vi "Begin.vi"(8 "error in":errorcluster) -> (0 "error out":errorcluster)   [LabVIEW 2019]
doc: "Called before other user functions, this VI is expected to open initial I/O refnums, load in file data, and do all program initialization. Notice that the <B>error out</B> terminal is simply used for data flow. Wiring it to other structures or subVIs ensures that this VI runs first."
uses:
  <vilib>/Rock Robotics/WPI/DriverStation/WPI_DriverStationRobotMode2.ctl
  <vilib>/Rock Robotics/WPI/Joystick/WPI_JoystickDeviceEnum.ctl
  <vilib>/Rock Robotics/SystemInterfaces/DIO/FPGA_DIOPWMChannel.ctl
  <vilib>/Rock Robotics/SystemInterfaces/DIO/FPGA_DIOChannel.ctl
  <vilib>/Rock Robotics/WPI/Solenoid/WPI_SolenoidChannel.ctl
  <vilib>/Rock Robotics/WPI/Accelerometer/WPI_AccelerometerAnalogChannels.ctl
  <vilib>/Rock Robotics/SystemInterfaces/AI/FPGA_AIChannel.ctl
  Robot Global Data.vi
  <vilib>/Rock Robotics/WPI/MotorControl/WPI_MotorControlOpen SPARK.vi
  <vilib>/Rock Robotics/WPI/Solenoid/WPI_SolenoidOpenDouble.vi
  <vilib>/Rock Robotics/WPI/Accelerometer/WPI_AccelerometerAnalogOpen.vi
  <vilib>/Rock Robotics/WPI/Switch/WPI_SwitchOpenLimit.vi
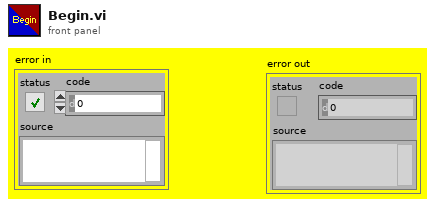
[diagram p1: front panel]
types:
  T1 = typedef "FPGA_DIOChannel.ctl" = enum8{"DIO 0", "DIO 1", "DIO 2", "DIO 3", "DIO 4", "DIO 5", "DIO 6", "DIO 7", "DIO 8", "DIO 9", "DIO MXP 0", "DIO MXP 1", "DIO MXP 2", "DIO MXP 3", "DIO MXP 4", "DIO MXP 5", "DIO MXP 6", "DIO MXP 7", "DIO MXP 8", "DIO MXP 9", "DIO MXP 10", "DIO MXP 11", "DIO MXP 12", "DIO MXP 13", "DIO MXP 14", "DIO MXP 15", "SPI Port CS1", "SPI Port CS2", "SPI Port CS3", "SPI Port MISO", "SPI Port MOSI", "Invalid"}
  T2 = typedef "FPGA_AIChannel.ctl" = enum8{"AI 0", "AI 1", "AI 2", "AI 3", "AI MXP 0", "AI MXP 1", "AI MXP 2", "AI MXP 3", "Invalid"}
  T3 = typedef "WPI_SolenoidChannel.ctl" = enum8{"Solenoid 0", "Solenoid 1", "Solenoid 2", "Solenoid 3", "Solenoid 4", "Solenoid 5", "Solenoid 6", "Solenoid 7", "Invalid"}
  T4 = typedef "WPI_AccelerometerAnalogChannels.ctl" = cluster{"X-Axis":T2, "Y-Axis":T2, "Z-Axis":T2}
  T5 = typedef "FPGA_DIOPWMChannel.ctl" = enum8{"PWM 0", "PWM 1", "PWM 2", "PWM 3", "PWM 4", "PWM 5", "PWM 6", "PWM 7", "PWM 8", "PWM 9", "PWM MXP 0", "PWM MXP 1", "PWM MXP 2", "PWM MXP 3", "PWM MXP 4", "PWM MXP 5", "PWM MXP 6", "PWM MXP 7", "PWM MXP 8", "PWM MXP 9", "Invalid"}
  T6 = typedef "WPI_JoystickDeviceEnum.ctl" = enum16{"USB 0", "USB 1", "USB 2", "USB 3", "USB 4", "USB 5"}
  T7 = typedef "WPI_DriverStationRobotMode2.ctl" = enum16{"Autonomous Disabled", "Autonomous Enabled", "Teleop Disabled", "Teleop Enabled", "Disconnected", "Finish", "Test Disabled", "Test Enabled", "Emergency Stopped"}
  T8 = typedef "WPI_JoystickDevRef.ctl" = cluster{"Device":T6}
  T9 = typedef "WPI_DigitalOutputDevRef.ctl" = cluster{"DIO Channel":T1, "DevStatus":errorcluster}
  T10 = typedef "WPI_MotorControlDeviceRef.ctl" = cluster{"DeviceStatus":errorcluster, "Type":T11, "PWM":cluster{"PWM Channel":T5, "DeadBand":T12}, "CAN":cluster{"Device Number":u8, "SetOutput VI Ref":variant, "GetOutput VI Ref":variant, "Enable VI Ref":variant, "Disable VI Ref":variant, "Data":variant}, "Invert":bool, "DIO PWM":cluster{"PWM \"Enable\" Channel":T5, "DIOChannel":T1, "PWM Rate":dbl}}
  T11 = typedef "WPI_MotorControlType.ctl" = enum16{"PWM", "CAN", "DIO PWM"}
  T12 = typedef "WPI_PWMDeadband.ctl" = cluster{"Name":string, "maxPositivePwm":i32, "minPositivePwm":i32, "centerPwm":i32, "maxNegativePwm":i32, "minNegativePwm":i32, "angularRange":u16}
  T13 = typedef "WPI_SolenoidDevRef.ctl" = cluster{"DevStatus":errorcluster, "Pneumatics Control Module":u8, "Forward Solenoid Channel":T3, "Reverse Solenoid Channel":T3}
  T14 = typedef "WPI_SwitchDevRef.ctl" = cluster{"DevStatus":errorcluster, "DIO Channel":T1, "CntIndex":T15, "Normally Closed":bool}
  T15 = typedef "FPGA_CounterCtrSystemIndex.ctl" = enum8{"Ctr 0", "Ctr 1", "Ctr 2", "Ctr 3", "Ctr 4", "Ctr 5", "Ctr 6", "Ctr 7", "Invalid"}
  T16 = typedef "WPI_PotentiometerDevRef.ctl" = cluster{"DevStatus":errorcluster, "Analog Channel":T2, "Invert Output":bool}
  T17 = typedef "WPI_AccelerometerDevRef.ctl" = cluster{"DevStatus":errorcluster, "Scaling":T18, "Analog Channels":T4, "I2C Bus":T19, "SPI Bus":T20, "Accel Range":T21, "ADXL Axes":T22, "Handle":i32, "Device Address":u8, "Accel Type":enum16{"Analog", "ADXL345 I2C", "ADXL345 SPI", "Internal", "ADXL362 SPI"}}
  T18 = typedef "WPI_AccelerometerScaling.ctl" = cluster{"Gain (VoltsPerG)":dbl, "Center Voltage":dbl}
  T19 = typedef "i2c_bus.ctl" = enum16{"I2C On-Board", "I2C MXP", "Invalid"}
  T20 = typedef "spi_bus.ctl" = enum16{"SPI On-Board, CS0", "SPI On-Board, CS1", "SPI On-Board, CS2", "SPI On-Board, CS3", "SPI MXP", "Invalid"}
  T21 = typedef "ADXL345 Range.ctl" = u8
  T22 = typedef "WPI_AccelerometerADXL345 Axes.ctl" = cluster{"X-Axis":bool, "Y-Axis":bool, "Z-Axis":bool}
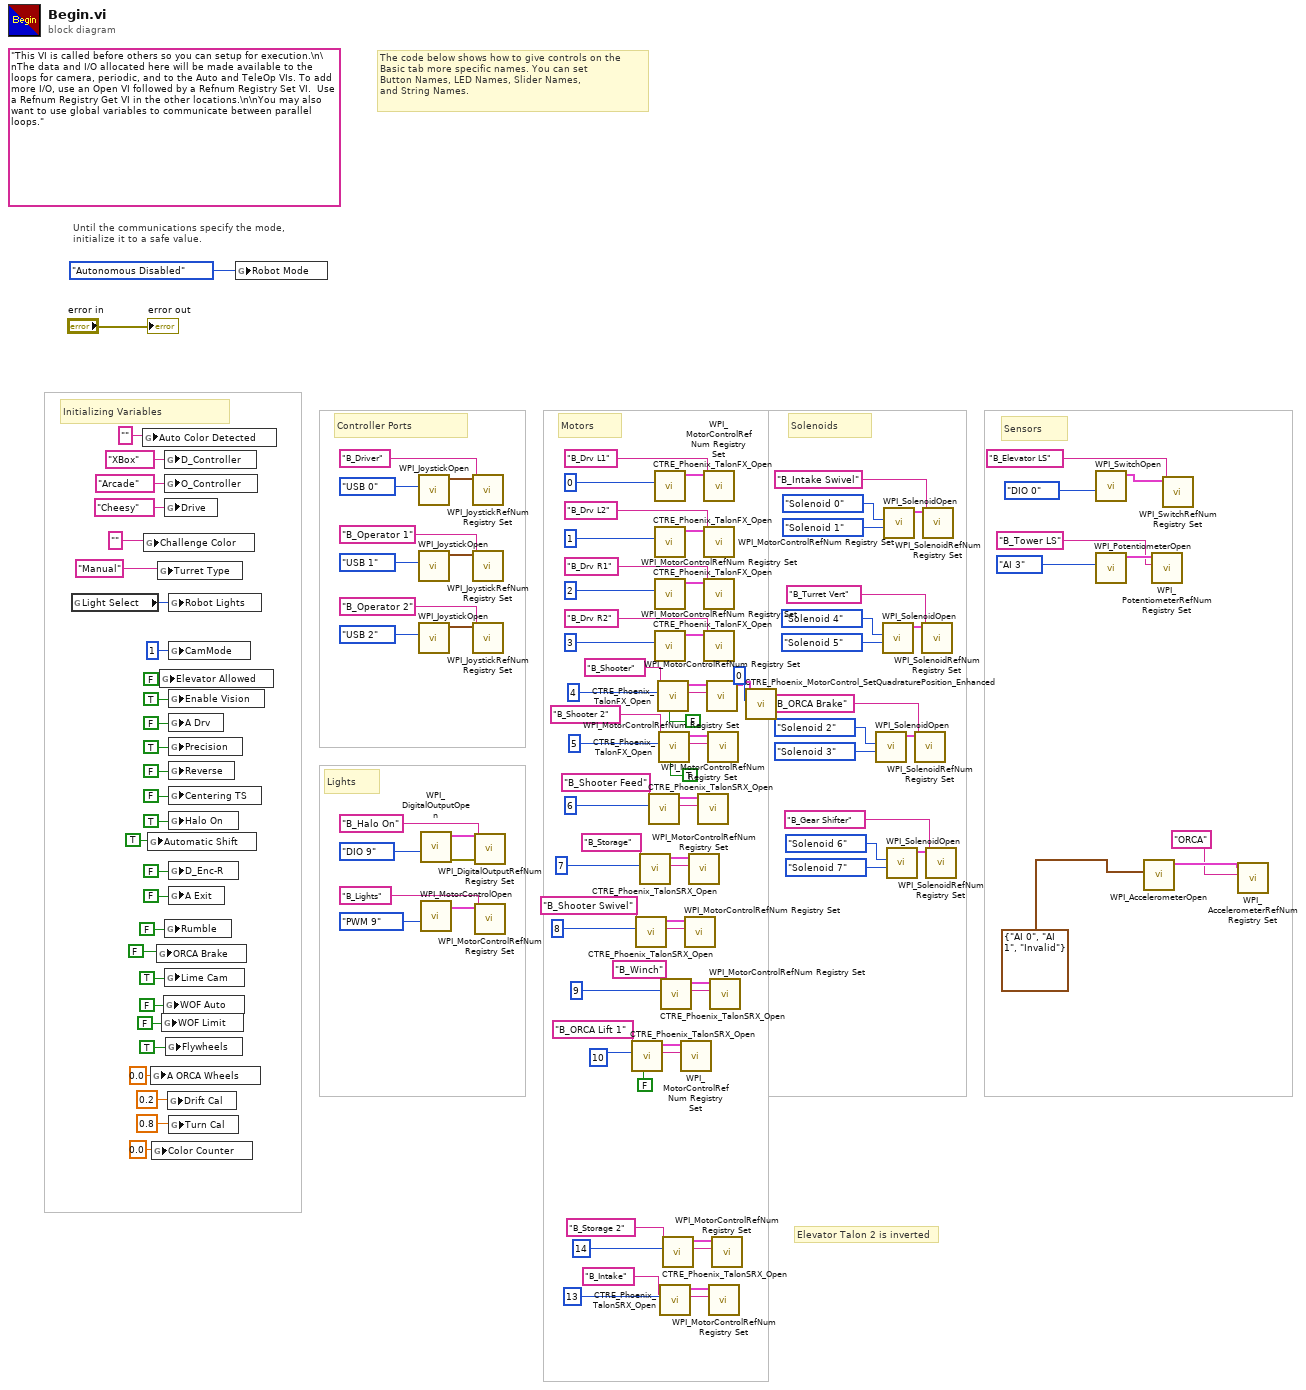
[diagram p0: block diagram]
diagram:
  (unwired) "This VI is called before others so you can setup for execution.\n\nThe data and I/O allocated here will be made available to the loops for camera, periodic, and to the Auto and TeleOp VIs. To add more I/O, use an Open VI followed by a Refnum Registry Set VI.  Use a Refnum Registry Get VI in the other locations.\n\nYou may also want to use global variables to communicate between parallel loops."
  # "Elevator Talon 2 is inverted"
  # "Sensors"
  # "Solenoids"
  # "Lights"
  # "Motors"
  # "Controller Ports"
  # "Initializing Variables"
  # "The code below shows how to give controls on the\nBasic tab more specific names. You can set\nButton Names, LED Names, Slider Names,\nand String Names."
  # "Until the communications specify the mode,\ninitialize it to a safe value."
  n1 = global read "Robot Global Data.vi" "Light Select"() -> (w99:i8)
  n2 = global write "Robot Global Data.vi" "Auto Color Detected"("" ("Auto Color Detected")) -> ()
  n3 = global write "Robot Global Data.vi" "Challenge Color"("" ("Auto Color Detected")) -> ()
  n4 = global write "Robot Global Data.vi" "Automatic Shift"(TRUE ("Enable Vision")) -> ()
  n5 = global write "Robot Global Data.vi" "A ORCA Wheels"(0.0 ("4Bar Dist")) -> ()
  n6 = global write "Robot Global Data.vi" "Color Counter"(0.0 ("Drift Cal")) -> ()
  n7 = global write "Robot Global Data.vi" "ORCA Brake"(FALSE ("ORCA Brake")) -> ()
  n8 = global write "Robot Global Data.vi" "Turret Type"("Manual" ("Auto Color Detected")) -> ()
  n9 = global write "Robot Global Data.vi" "Elevator Allowed"(FALSE ("Enable Vision")) -> ()
  n10 = global write "Robot Global Data.vi" "WOF Limit"(FALSE ("Enable Vision")) -> ()
  n11 = global write "Robot Global Data.vi" "WOF Auto"(FALSE ("Enable Vision")) -> ()
  n12 = global write "Robot Global Data.vi" "D_Controller"("XBox" ("D_Controller")) -> ()
  n13 = global write "Robot Global Data.vi" "O_Controller"("Arcade" ("O_Controller")) -> ()
  n14 = global write "Robot Global Data.vi" "Drive"("Cheesy" ("Drive")) -> ()
  n15 = global write "Robot Global Data.vi" "Rumble"(FALSE ("Enable Vision")) -> ()
  n16 = global write "Robot Global Data.vi" "Lime Cam"(TRUE ("Enable Vision")) -> ()
  n17 = global write "Robot Global Data.vi" "Flywheels"(TRUE ("Enable Vision")) -> ()
  n18 = global write "Robot Global Data.vi" "Drift Cal"(0.2 ("Drift Cal")) -> ()
  n19 = global write "Robot Global Data.vi" "Robot Lights"(w99) -> ()
  n20 = global write "Robot Global Data.vi" "CamMode"(i8 1 ("Light Select")) -> ()
  n21 = global write "Robot Global Data.vi" "Enable Vision"(TRUE ("Enable Vision")) -> ()
  n22 = global write "Robot Global Data.vi" "A Drv"(FALSE ("Enable Vision")) -> ()
  n23 = global write "Robot Global Data.vi" "Precision"(TRUE ("Enable Vision")) -> ()
  n24 = global write "Robot Global Data.vi" "Reverse"(FALSE ("Enable Vision")) -> ()
  n25 = global write "Robot Global Data.vi" "Centering TS"(FALSE ("Enable Vision")) -> ()
  n26 = global write "Robot Global Data.vi" "Halo On"(TRUE ("Enable Vision")) -> ()
  n27 = global write "Robot Global Data.vi" "D_Enc-R"(FALSE ("Enable Vision")) -> ()
  n28 = global write "Robot Global Data.vi" "A Exit"(FALSE ("Enable Vision")) -> ()
  n29 = global write "Robot Global Data.vi" "Turn Cal"(0.8 ("Drift Cal")) -> ()
  n30 = global write "Robot Global Data.vi" "Robot Mode"(WPI_DriverStationRobotMode2."Autonomous Disabled" ("Robot Mode")) -> ()
  n31 = call <vilib>:"WPI_JoystickOpen.vi"("JoystickDevice"=WPI_JoystickDeviceEnum."USB 0") -> ("JoystickDevRef"=w86:T8)  [unwired: 10 in]
  n32 = call <vilib>:"WPI_JoystickOpen.vi"("JoystickDevice"=WPI_JoystickDeviceEnum."USB 1") -> ("JoystickDevRef"=w83:T8)  [unwired: 10 in]
  n33 = call <vilib>:"WPI_JoystickOpen.vi"("JoystickDevice"=WPI_JoystickDeviceEnum."USB 2") -> ("JoystickDevRef"=w81:T8)  [unwired: 10 in]
  n34 = call <vilib>:"WPI_DigitalOutputOpen.vi"("DIO Channel"=FPGA_DIOChannel."DIO 9") -> ("error out"=w62:errorcluster, "DigitalOutputDevRef"=w61:T9)  [unwired: 9 in]
  n35 = call-poly <vilib>:"WPI_MotorControlOpen.vi"("PWM Channel"=FPGA_DIOPWMChannel."PWM 9") -> ("MotorControlDeviceRef"=w64:T10)  [unwired: 9 in, 1 out]
  n36 = call <vilib>:"WPI_JoystickRefNum Registry Set.vi"("refnum name"="B_Driver", "JoystickDevRef"=w86) -> ()  [unwired: 8 in, 2 out]
  n37 = call <vilib>:"WPI_JoystickRefNum Registry Set.vi"("refnum name"="B_Operator 1", "JoystickDevRef"=w83) -> ()  [unwired: 8 in, 2 out]
  n38 = call <vilib>:"WPI_JoystickRefNum Registry Set.vi"("refnum name"="B_Operator 2", "JoystickDevRef"=w81) -> ()  [unwired: 8 in, 2 out]
  n39 = call <vilib>:"WPI_DigitalOutputRefNum Registry Set.vi"("error in (no error)"=w62, "refnum name"="B_Halo On", "DigitalOutputDevRef"=w61) -> ()  [unwired: 7 in, 2 out]
  n40 = call <vilib>:"WPI_MotorControlRefNum Registry Set.vi"("refnum name"="B_Lights", "MotorControlDevRef"=w64) -> ()  [unwired: 8 in, 2 out]
  n41 = call <vilib>:"CTRE_Phoenix_TalonSRX_Open.vi"("Invert"=FALSE, "Device Number"=u8 10) -> ("CAN Talon SRX Ref"=w52:T10)  [unwired: 8 in, 1 out]
  n42 = call <vilib>:"CTRE_Phoenix_TalonSRX_Open.vi"("Device Number"=u8 8) -> ("CAN Talon SRX Ref"=w27:T10)  [unwired: 9 in, 1 out]
  n43 = call <vilib>:"CTRE_Phoenix_TalonSRX_Open.vi"("Device Number"=u8 7) -> ("CAN Talon SRX Ref"=w21:T10)  [unwired: 9 in, 1 out]
  n44 = call <vilib>:"CTRE_Phoenix_TalonSRX_Open.vi"("Device Number"=u8 6) -> ("CAN Talon SRX Ref"=w24:T10)  [unwired: 9 in, 1 out]
  n45 = call <vilib>:"CTRE_Phoenix_TalonFX_Open.vi"("Device Number"=u8 0) -> ("CAN Talon SRX Ref"=w76:T10)  [unwired: 9 in, 1 out]
  n46 = call <vilib>:"CTRE_Phoenix_TalonFX_Open.vi"("Device Number"=u8 1) -> ("CAN Talon SRX Ref"=w67:T10)  [unwired: 9 in, 1 out]
  n47 = call <vilib>:"CTRE_Phoenix_TalonFX_Open.vi"("Device Number"=u8 2) -> ("CAN Talon SRX Ref"=w73:T10)  [unwired: 9 in, 1 out]
  n48 = call <vilib>:"CTRE_Phoenix_TalonFX_Open.vi"("Device Number"=u8 3) -> ("CAN Talon SRX Ref"=w70:T10)  [unwired: 9 in, 1 out]
  n49 = call <vilib>:"CTRE_Phoenix_TalonFX_Open.vi"("Invert"=FALSE, "Device Number"=u8 4) -> ("CAN Talon SRX Ref"=w51:T10)  [unwired: 8 in, 1 out]
  n50 = call <vilib>:"CTRE_Phoenix_TalonFX_Open.vi"("Invert"=TRUE, "Device Number"=u8 5) -> ("CAN Talon SRX Ref"=w49:T10)  [unwired: 8 in, 1 out]
  n51 = call <vilib>:"CTRE_Phoenix_TalonSRX_Open.vi"("Device Number"=u8 13) -> ("CAN Talon SRX Ref"=w58:T10)  [unwired: 9 in, 1 out]
  n52 = call <vilib>:"CTRE_Phoenix_TalonSRX_Open.vi"("Device Number"=u8 9) -> ("CAN Talon SRX Ref"=w53:T10)  [unwired: 9 in, 1 out]
  n53 = call <vilib>:"CTRE_Phoenix_TalonSRX_Open.vi"("Device Number"=u8 14) -> ("CAN Talon SRX Ref"=w18:T10)  [unwired: 9 in, 1 out]
  n54 = call <vilib>:"WPI_MotorControlRefNum Registry Set.vi"("refnum name"="B_ORCA Lift 1", "MotorControlDevRef"=w52) -> ()  [unwired: 8 in, 2 out]
  n55 = call <vilib>:"WPI_MotorControlRefNum Registry Set.vi"("refnum name"="B_Shooter Swivel", "MotorControlDevRef"=w27) -> ()  [unwired: 8 in, 2 out]
  n56 = call <vilib>:"WPI_MotorControlRefNum Registry Set.vi"("refnum name"="B_Storage", "MotorControlDevRef"=w21) -> ()  [unwired: 8 in, 2 out]
  n57 = call <vilib>:"WPI_MotorControlRefNum Registry Set.vi"("refnum name"="B_Shooter Feed", "MotorControlDevRef"=w24) -> ()  [unwired: 8 in, 2 out]
  n58 = call <vilib>:"WPI_MotorControlRefNum Registry Set.vi"("refnum name"="B_Drv L1", "MotorControlDevRef"=w76) -> ()  [unwired: 8 in, 2 out]
  n59 = call <vilib>:"WPI_MotorControlRefNum Registry Set.vi"("refnum name"="B_Drv L2", "MotorControlDevRef"=w67) -> ()  [unwired: 8 in, 2 out]
  n60 = call <vilib>:"WPI_MotorControlRefNum Registry Set.vi"("refnum name"="B_Drv R1", "MotorControlDevRef"=w73) -> ()  [unwired: 8 in, 2 out]
  n61 = call <vilib>:"WPI_MotorControlRefNum Registry Set.vi"("refnum name"="B_Drv R2", "MotorControlDevRef"=w70) -> ()  [unwired: 8 in, 2 out]
  n62 = call <vilib>:"WPI_MotorControlRefNum Registry Set.vi"("refnum name"="B_Shooter", "MotorControlDevRef"=w51) -> ("MotorControlDevRef"=w1:T10)  [unwired: 8 in, 1 out]
  n63 = call <vilib>:"WPI_MotorControlRefNum Registry Set.vi"("refnum name"="B_Shooter 2", "MotorControlDevRef"=w49) -> ()  [unwired: 8 in, 2 out]
  n64 = call <vilib>:"WPI_MotorControlRefNum Registry Set.vi"("refnum name"="B_Intake", "MotorControlDevRef"=w58) -> ()  [unwired: 8 in, 2 out]
  n65 = call <vilib>:"WPI_MotorControlRefNum Registry Set.vi"("refnum name"="B_Winch", "MotorControlDevRef"=w53) -> ()  [unwired: 8 in, 2 out]
  n66 = call <vilib>:"WPI_MotorControlRefNum Registry Set.vi"("refnum name"="B_Storage 2", "MotorControlDevRef"=w18) -> ()  [unwired: 8 in, 2 out]
  n67 = call <vilib>:"CTRE_Phoenix_MotorControl_SetQuadraturePosition_Enhanced.vi"("New Position"=0, "PhoenixMotorControlDevRef"=w1) -> ()  [unwired: 8 in, 2 out]
  n68 = call-poly <vilib>:"WPI_SolenoidOpen.vi"("Reverse Solenoid Channel"=WPI_SolenoidChannel."Solenoid 3", "Forward Solenoid Channel"=WPI_SolenoidChannel."Solenoid 2") -> ("SolenoidDevRef"=w48:T13)  [unwired: 8 in, 1 out]
  n69 = call-poly <vilib>:"WPI_SolenoidOpen.vi"("Reverse Solenoid Channel"=WPI_SolenoidChannel."Solenoid 5", "Forward Solenoid Channel"=WPI_SolenoidChannel."Solenoid 4") -> ("SolenoidDevRef"=w16:T13)  [unwired: 8 in, 1 out]
  n70 = call-poly <vilib>:"WPI_SolenoidOpen.vi"("Reverse Solenoid Channel"=WPI_SolenoidChannel."Solenoid 1", "Forward Solenoid Channel"=WPI_SolenoidChannel."Solenoid 0") -> ("SolenoidDevRef"=w38:T13)  [unwired: 8 in, 1 out]
  n71 = call-poly <vilib>:"WPI_SolenoidOpen.vi"("Reverse Solenoid Channel"=WPI_SolenoidChannel."Solenoid 7", "Forward Solenoid Channel"=WPI_SolenoidChannel."Solenoid 6") -> ("SolenoidDevRef"=w29:T13)  [unwired: 8 in, 1 out]
  n72 = call <vilib>:"WPI_SolenoidRefNum Registry Set.vi"("refnum name"="B_ORCA Brake", "SolenoidDevRef"=w48) -> ()  [unwired: 8 in, 2 out]
  n73 = call <vilib>:"WPI_SolenoidRefNum Registry Set.vi"("refnum name"="B_Turret Vert", "SolenoidDevRef"=w16) -> ()  [unwired: 8 in, 2 out]
  n74 = call <vilib>:"WPI_SolenoidRefNum Registry Set.vi"("refnum name"="B_Intake Swivel", "SolenoidDevRef"=w38) -> ()  [unwired: 8 in, 2 out]
  n75 = call <vilib>:"WPI_SolenoidRefNum Registry Set.vi"("refnum name"="B_Gear Shifter", "SolenoidDevRef"=w29) -> ()  [unwired: 8 in, 2 out]
  n76 = call-poly <vilib>:"WPI_SwitchOpen.vi"("DIO Channel"=FPGA_DIOChannel."DIO 0") -> ("SwitchDevRef"=w4:T14)  [unwired: 9 in, 1 out]
  n77 = call <vilib>:"WPI_PotentiometerOpen.vi"("Analog Channel"=FPGA_AIChannel."AI 3") -> ("PotDevRef"=w12:T16)  [unwired: 9 in, 1 out]
  n78 = call-poly <vilib>:"WPI_AccelerometerOpen.vi"("Analog Channels"=T4 {"X-Axis"=enum."AI 0", "Y-Axis"=enum."AI 1", "Z-Axis"=enum."Invalid"}) -> ("AccelerometerDevRef"=w44:T17)  [unwired: 9 in, 1 out]
  n79 = call <vilib>:"WPI_PotentiometerRefNum Registry Set.vi"("refnum name"="B_Tower LS", "PotDevRef"=w12) -> ()  [unwired: 8 in, 2 out]
  n80 = call <vilib>:"WPI_SwitchRefNum Registry Set.vi"("refnum name"="B_Elevator LS", "SwitchDevRef"=w4) -> ()  [unwired: 8 in, 2 out]
  n81 = call <vilib>:"WPI_AccelerometerRefNum Registry Set.vi"("refnum name"="ORCA", "AccelerometerDevRef"=w44) -> ()  [unwired: 8 in, 2 out]
  "error out" <- "error in"
